vi "Initialize Message Log.vi"(8 "error in (no error)":errorcluster) -> (0 "error out":errorcluster)   [LabVIEW 2015, in "UI Handler.lvclass"]
uses:
  UI Handler.lvclass
  UI Handler.lvclass/UI Handler.ctl
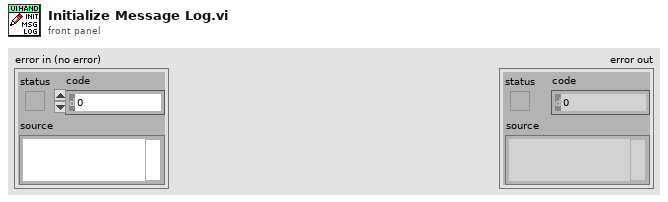
[diagram p1: front panel]
types:
  T1 = typedef "UI Handler.lvclass/Session Handle.ctl" = refnum<data-value>
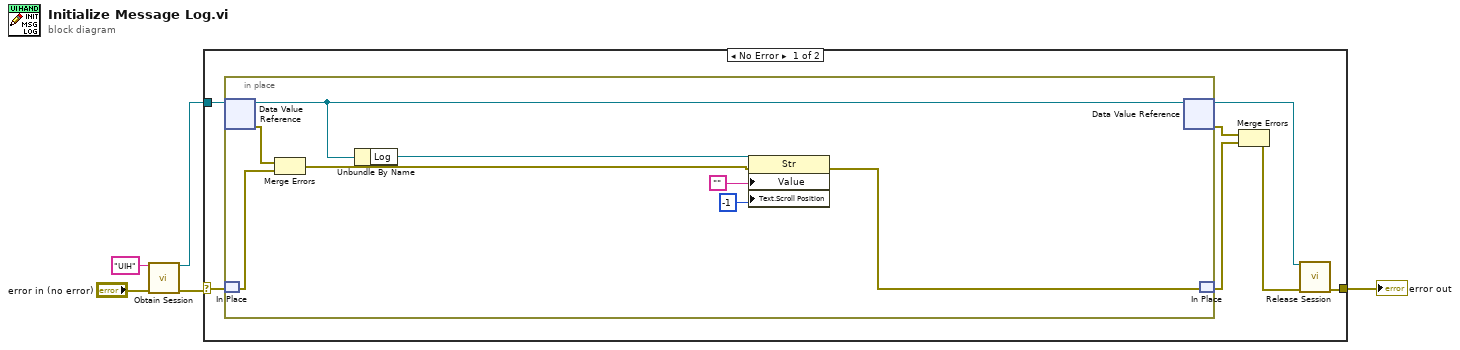
[diagram p0: block diagram]
diagram:
  n1 = call "Obtain Session.vi"("Session  Name ()"="UIH", "error in (no error)"="error in (no error)") -> ("Session Handle"=w1:T1, "error out"=w2:errorcluster)  [unwired: 12 in]
  n2 = case shown="No Error" w2 {
    selector: w2 -> [w9 w21]
    tunnel: w1 -> [w12 _]
    tunnel: [w7 w21] -> w4
    frame No Error {
      n3 = in-place {
        n4 = in-place-dvr #1(w12) -> (w20:refnum<class "UI Handler.lvclass">, w18:errorcluster)
        n5 = in-place-match #2(w9) -> (w17:errorcluster)
        n6 = Merge Errors(w18, w17) -> (w13:errorcluster)
        n7 = Unbundle By Name(w20) -> ("Log"=w15:refnum<vi>)
        n8 = property class="Str"(reference=w15, error in=w13, "Value"="", "Text.Scroll Position"=-1) -> (error out=w16:errorcluster)  [unwired: 1 out]
        n9 = in-place-dvr #1(w20) -> (w6:T1, w10:errorcluster)
        n10 = in-place-match #2(w16) -> (w11:errorcluster)
      }
      n11 = Merge Errors(w10, w11) -> (w8:errorcluster)
      n12 = call "Release Session.vi"("Session Handle"=w6, "error in (no error)"=w8) -> ("error out"=w7:errorcluster)  [unwired: 13 in]
    }
    frame Error {
    }
  }
  "error out" <- w4
